vi "Flow_Commands.vi"(1 "Debug Mode":bool, 2 "Flow Array":dbl[](array[numeric]), 3 "Command":string) -> ()   [LabVIEW 2011]
doc: "This VI executes all gas flow commands. It uses the supplied flow array, with indicies 0, 1, 2, and 3 correlating to Flows 1, 2, 3 and 4 for a given gas on the MOCVD front panel. All supplied values should be in units of sccm. This VI will make the applicable voltage calculations and send them to the required slots and channels HP 6940B multiprogrammer. Debug mode disables all hardware communication functionality."
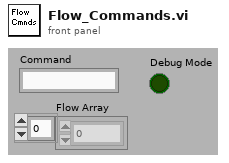
[diagram p1: front panel]
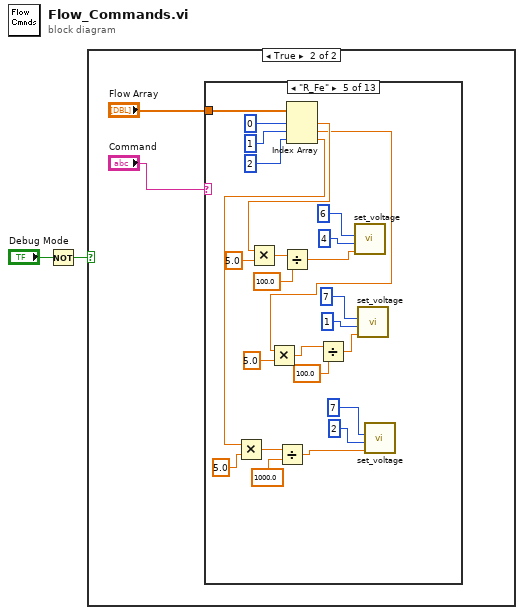
[diagram p0: block diagram]
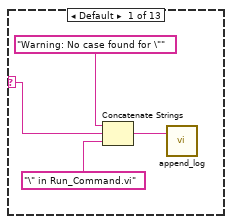
[diagram p3: hidden frame]
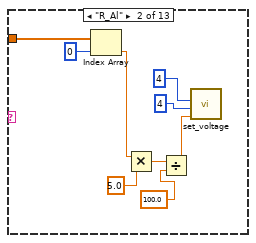
[diagram p4: hidden frame]
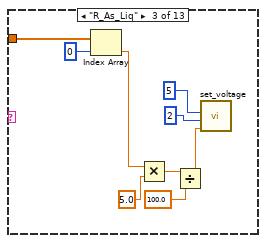
[diagram p5: hidden frame]
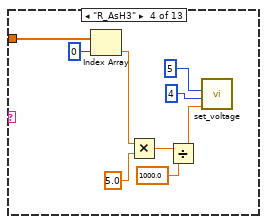
[diagram p6: hidden frame]
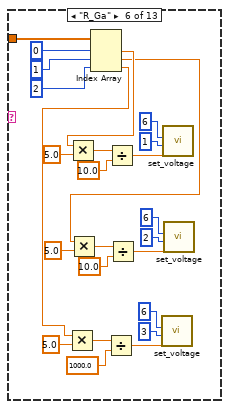
[diagram p7: hidden frame]
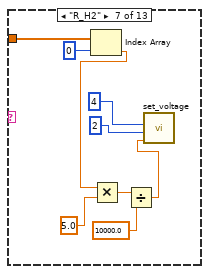
[diagram p8: hidden frame]
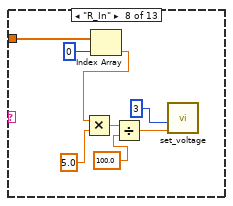
[diagram p9: hidden frame]
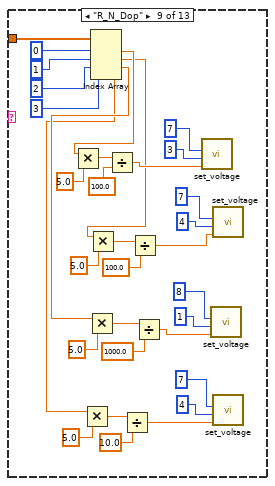
[diagram p10: hidden frame]
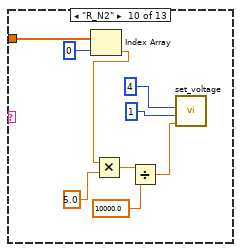
[diagram p11: hidden frame]
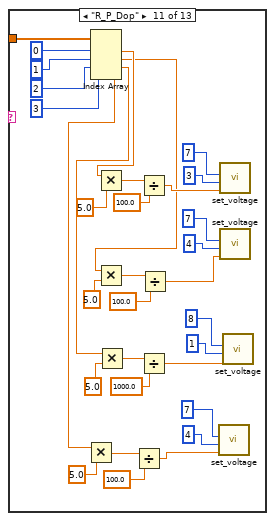
[diagram p12: hidden frame]
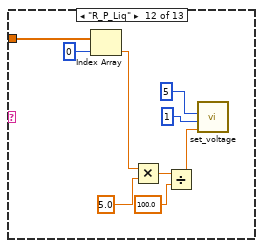
[diagram p13: hidden frame]
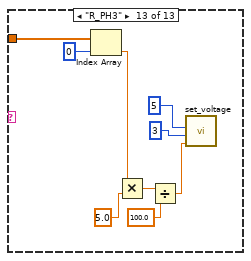
[diagram p14: hidden frame]
diagram:
  n1 = Not(x="Debug Mode") -> (.not. x?=w2:bool)
  n2 = case shown="True" w2 {
    frame False {
    }
    frame True {
      n3 = case shown="\"R_Fe\"" "Command" {
        selector: "Command" -> [w7 _ _ _ _ _ _ _ _ _ _ _ _]
        tunnel: "Flow Array" -> [_ w17 w26 w35 w60 w85 w94 w102 w135 w144 w177 w186 w195]
        frame Default {
          n4 = Concatenate Strings("Warning: No case found for \"" ("message"), w7, "\" in Run_Command.vi" ("string")) -> (w5:string)
          n5 = call "append_log.vi"("New Log String"=w5) -> ()  [unwired: 1 in, 1 out]
        }
        frame "R_Al" {
          n6 = Index Array(array=w17, index=0) -> (element=w9:dbl)
          n7 = Multiply(x=w9, y=5.0) -> (x*y=w13:dbl)
          n8 = Divide(x=w13, y=100.0) -> (x/y=w11:dbl)
          n9 = call "set_voltage.vi"("Voltage"=w11, "Channel"=4, "Slot"=4) -> ()  [unwired: 1 in, 1 out]
        }
        frame "R_As_Liq" {
          n10 = Index Array(array=w26, index=0) -> (element=w18:dbl)
          n11 = Multiply(x=w18, y=5.0) -> (x*y=w21:dbl)
          n12 = Divide(x=w21, y=100.0) -> (x/y=w19:dbl)
          n13 = call "set_voltage.vi"("Voltage"=w19, "Channel"=2, "Slot"=5) -> ()  [unwired: 1 in, 1 out]
        }
        frame "R_AsH3" {
          n14 = Index Array(array=w35, index=0) -> (element=w27:dbl)
          n15 = Multiply(x=w27, y=5.0) -> (x*y=w30:dbl)
          n16 = Divide(x=w30, y=1000.0) -> (x/y=w28:dbl)
          n17 = call "set_voltage.vi"("Voltage"=w28, "Channel"=4, "Slot"=5) -> ()  [unwired: 1 in, 1 out]
        }
        frame "R_Fe" {
          n18 = Index Array(array=w60, index #1=0 ("index"), index #2=1 ("index"), index #3=2 ("index")) -> (element #1=w50:dbl, element #2=w37:dbl, element #3=w36:dbl)
          n19 = Multiply(x=w36, y=5.0) -> (x*y=w40:dbl)
          n20 = Multiply(x=w50, y=5.0) -> (x*y=w54:dbl)
          n21 = Multiply(x=w37, y=5.0) -> (x*y=w46:dbl)
          n22 = Divide(x=w40, y=1000.0) -> (x/y=w38:dbl)
          n23 = Divide(x=w54, y=100.0) -> (x/y=w56:dbl)
          n24 = Divide(x=w46, y=100.0) -> (x/y=w44:dbl)
          n25 = call "set_voltage.vi"("Voltage"=w56, "Channel"=4, "Slot"=6) -> ()  [unwired: 1 in, 1 out]
          n26 = call "set_voltage.vi"("Voltage"=w44, "Channel"=1, "Slot"=7) -> ()  [unwired: 1 in, 1 out]
          n27 = call "set_voltage.vi"("Voltage"=w38, "Channel"=2, "Slot"=7) -> ()  [unwired: 1 in, 1 out]
        }
        frame "R_Ga" {
          n28 = Index Array(array=w85, index #1=0 ("index"), index #2=1 ("index"), index #3=2 ("index")) -> (element #1=w75:dbl, element #2=w68:dbl, element #3=w61:dbl)
          n29 = Multiply(x=w61, y=5.0) -> (x*y=w65:dbl)
          n30 = Multiply(x=w75, y=5.0) -> (x*y=w79:dbl)
          n31 = Multiply(x=w68, y=5.0) -> (x*y=w72:dbl)
          n32 = Divide(x=w65, y=1000.0) -> (x/y=w67:dbl)
          n33 = Divide(x=w79, y=10.0) -> (x/y=w81:dbl)
          n34 = Divide(x=w72, y=10.0) -> (x/y=w74:dbl)
          n35 = call "set_voltage.vi"("Voltage"=w67, "Channel"=3, "Slot"=6) -> ()  [unwired: 1 in, 1 out]
          n36 = call "set_voltage.vi"("Voltage"=w81, "Channel"=1, "Slot"=6) -> ()  [unwired: 1 in, 1 out]
          n37 = call "set_voltage.vi"("Voltage"=w74, "Channel"=2, "Slot"=6) -> ()  [unwired: 1 in, 1 out]
        }
        frame "R_H2" {
          n38 = Index Array(array=w94, index=0) -> (element=w86:dbl)
          n39 = Multiply(x=w86, y=5.0) -> (x*y=w88:dbl)
          n40 = Divide(x=w88, y=10000.0) -> (x/y=w90:dbl)
          n41 = call "set_voltage.vi"("Voltage"=w90, "Channel"=2, "Slot"=4) -> ()  [unwired: 1 in, 1 out]
        }
        frame "R_In" {
          n42 = Index Array(array=w102, index=0) -> (element=w95:dbl)
          n43 = Multiply(x=w95, y=5.0) -> (x*y=w98:dbl)
          n44 = Divide(x=w98, y=100.0) -> (x/y=w100:dbl)
          n45 = call "set_voltage.vi"("Voltage"=w100, "Channel"=3) -> ()  [unwired: 2 in, 1 out]
        }
        frame "R_N_Dop" {
          n46 = Index Array(array=w135, index #1=0 ("index"), index #2=1 ("index"), index #3=2 ("index"), index #4=3 ("index")) -> (element #1=w124:dbl, element #2=w117:dbl, element #3=w110:dbl, element #4=w103:dbl)
          n47 = Multiply(x=w124, y=5.0) -> (x*y=w128:dbl)
          n48 = Multiply(x=w103, y=5.0) -> (x*y=w107:dbl)
          n49 = Multiply(x=w110, y=5.0) -> (x*y=w114:dbl)
          n50 = Multiply(x=w117, y=5.0) -> (x*y=w121:dbl)
          n51 = Divide(x=w128, y=100.0) -> (x/y=w130:dbl)
          n52 = Divide(x=w107, y=10.0) -> (x/y=w109:dbl)
          n53 = Divide(x=w121, y=100.0) -> (x/y=w123:dbl)
          n54 = Divide(x=w114, y=1000.0) -> (x/y=w116:dbl)
          n55 = call "set_voltage.vi"("Voltage"=w130, "Channel"=3, "Slot"=7) -> ()  [unwired: 1 in, 1 out]
          n56 = call "set_voltage.vi"("Voltage"=w116, "Channel"=1, "Slot"=8) -> ()  [unwired: 1 in, 1 out]
          n57 = call "set_voltage.vi"("Voltage"=w123, "Channel"=4, "Slot"=7) -> ()  [unwired: 1 in, 1 out]
          n58 = call "set_voltage.vi"("Voltage"=w109, "Channel"=4, "Slot"=7) -> ()  [unwired: 1 in, 1 out]
        }
        frame "R_N2" {
          n59 = Index Array(array=w144, index=0) -> (element=w136:dbl)
          n60 = Multiply(x=w136, y=5.0) -> (x*y=w138:dbl)
          n61 = Divide(x=w138, y=10000.0) -> (x/y=w142:dbl)
          n62 = call "set_voltage.vi"("Voltage"=w142, "Channel"=1, "Slot"=4) -> ()  [unwired: 1 in, 1 out]
        }
        frame "R_P_Dop" {
          n63 = Index Array(array=w177, index #1=0 ("index"), index #2=1 ("index"), index #3=2 ("index"), index #4=3 ("index")) -> (element #1=w166:dbl, element #2=w159:dbl, element #3=w152:dbl, element #4=w145:dbl)
          n64 = Multiply(x=w145, y=5.0) -> (x*y=w149:dbl)
          n65 = Multiply(x=w166, y=5.0) -> (x*y=w170:dbl)
          n66 = Multiply(x=w159, y=5.0) -> (x*y=w160:dbl)
          n67 = Multiply(x=w152, y=5.0) -> (x*y=w156:dbl)
          n68 = Divide(x=w149, y=100.0) -> (x/y=w151:dbl)
          n69 = Divide(x=w170, y=100.0) -> (x/y=w172:dbl)
          n70 = Divide(x=w156, y=1000.0) -> (x/y=w158:dbl)
          n71 = Divide(x=w160, y=100.0) -> (x/y=w165:dbl)
          n72 = call "set_voltage.vi"("Voltage"=w151, "Channel"=4, "Slot"=7) -> ()  [unwired: 1 in, 1 out]
          n73 = call "set_voltage.vi"("Voltage"=w172, "Channel"=3, "Slot"=7) -> ()  [unwired: 1 in, 1 out]
          n74 = call "set_voltage.vi"("Voltage"=w165, "Channel"=4, "Slot"=7) -> ()  [unwired: 1 in, 1 out]
          n75 = call "set_voltage.vi"("Voltage"=w158, "Channel"=1, "Slot"=8) -> ()  [unwired: 1 in, 1 out]
        }
        frame "R_P_Liq" {
          n76 = Index Array(array=w186, index=0) -> (element=w178:dbl)
          n77 = Multiply(x=w178, y=5.0) -> (x*y=w182:dbl)
          n78 = Divide(x=w182, y=100.0) -> (x/y=w184:dbl)
          n79 = call "set_voltage.vi"("Voltage"=w184, "Channel"=1, "Slot"=5) -> ()  [unwired: 1 in, 1 out]
        }
        frame "R_PH3" {
          n80 = Index Array(array=w195, index=0) -> (element=w187:dbl)
          n81 = Multiply(x=w187, y=5.0) -> (x*y=w191:dbl)
          n82 = Divide(x=w191, y=100.0) -> (x/y=w193:dbl)
          n83 = call "set_voltage.vi"("Voltage"=w193, "Channel"=3, "Slot"=5) -> ()  [unwired: 1 in, 1 out]
        }
      }
    }
  }
